vi "LL to Dist.vi"(11 "limelightV":dbl) -> (3 "distance":dbl)   [LabVIEW 2020]
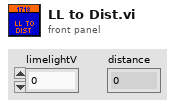
[diagram p1: front panel]
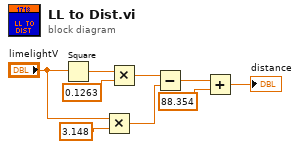
[diagram p0: block diagram]
diagram:
  n1 = Square(x="limelightV") -> (x^2=w9:dbl)
  n2 = Multiply(x="limelightV", y=3.148) -> (x*y=w4:dbl)
  n3 = Multiply(x=w9, y=0.1263) -> (x*y=w7:dbl)
  n4 = Subtract(x=w7, y=w4) -> (x-y=w3:dbl)
  n5 = Add(x=w3, y=88.354) -> (x+y=→"distance":dbl)
